vi "Untitled 1.vi"() -> ()   [LabVIEW 2021, in "FFT.lvlib"]
uses:
  FFT.lvlib
  <vilib>/Analysis/4window.llb/Hanning Window (DBL).vi
  <vilib>/Analysis/5stat.llb/RMS (DBL).vi
  <vilib>/Analysis/2dsp.llb/Real FFT.vi
  <vilib>/Analysis/4window.llb/AllCosWindow (DBL).vi
  <vilib>/Analysis/NI_AALPro.lvlib
panel:
  out "ACC Data":dbl[](array[numeric])
  out "Frequency measured":dbl
  out "FFT":dbl[](array[numeric])
  out "Low-Energy Warning":bool
  in  "Bound to 1st Frequency":bool=TRUE
  in  "Experiment":T1
  in  "Accelerometer sample":dbl[](array[numeric])
  in  "Frequency Method":T2(ring)
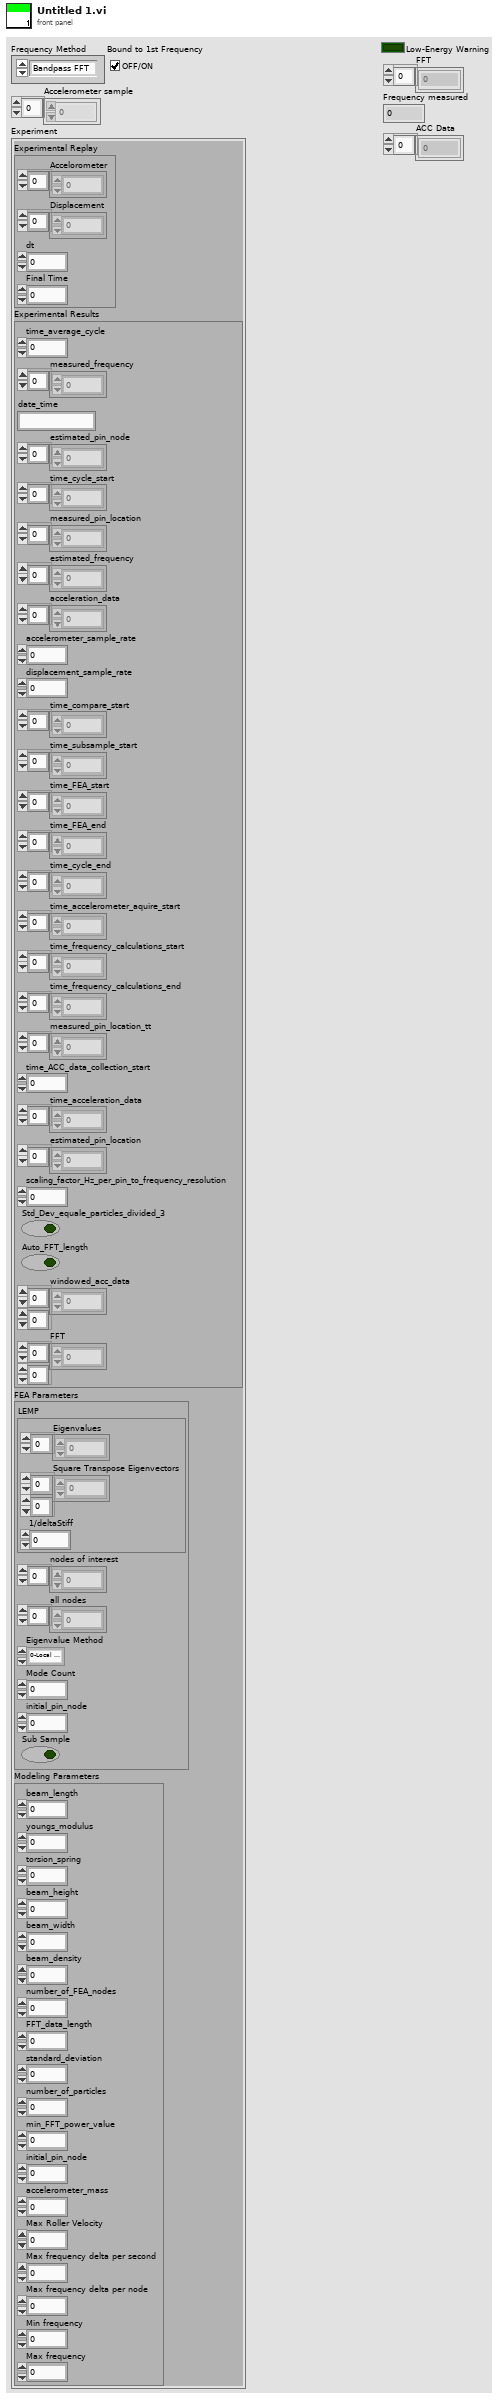
[diagram p1: front panel]
types:
  T1 = cluster{"Experimental Replay":cluster{"Accelorometer":dbl[], "Displacement":dbl[], "dt":dbl, "Final Time":dbl}, "Experimental Results":cluster{"time_average_cycle":dbl, "measured_frequency":dbl[], "date_time":string, "estimated_pin_node":i32[], "time_cycle_start":dbl[], "measured_pin_location":dbl[], "estimated_frequency":dbl[], "acceleration_data":dbl[], "accelerometer_sample_rate":dbl, "displacement_sample_rate":dbl, "time_compare_start":dbl[], "time_subsample_start":dbl[], "time_FEA_start":dbl[], "time_FEA_end":dbl[], "time_cycle_end":dbl[], "time_accelerometer_aquire_start":dbl[], "time_frequency_calculations_start":dbl[], "time_frequency_calculations_end":dbl[], "measured_pin_location_tt":dbl[], "time_ACC_data_collection_start":dbl, "time_acceleration_data":dbl[], "estimated_pin_location":dbl[], "scaling_factor_Hz_per_pin_to_frequency_resolution":dbl, "Std_Dev_equale_particles_divided_3":bool, "Auto_FFT_length":bool, "windowed_acc_data":dbl[][], "FFT":dbl[][]}, "FEA Parameters":cluster{"LEMP":cluster{"Eigenvalues":dbl[], "Square Transpose Eigenvectors":dbl[][], "1/deltaStiff":dbl}, "nodes of interest":i32[], "all nodes":i32[], "Eigenvalue Method":enum16{"0-Local Eigen Modification Procedure", "1-LabVIEW generalized eigenvalues", "2-LabVIEW M^-1K eigenvalues", "3-LabVIEW Cholesky Factorization", "4-Cholesky Factorization CPU SGL", "5-Cholesky Factorization CPU FXP", "6-Cholesky Factorization FPGA SGL", "7-Cholesky Factorization FPGA SGL SCL"}, "Mode Count":i32, "initial_pin_node":i32, "Sub Sample":bool}, "Modeling Parameters":cluster{"beam_length":dbl, "youngs_modulus":dbl, "torsion_spring":dbl, "beam_height":dbl, "beam_width":dbl, "beam_density":dbl, "number_of_FEA_nodes":i32, "FFT_data_length":i32, "standard_deviation":dbl, "number_of_particles":i32, "min_FFT_power_value":dbl, "initial_pin_node":i32, "accelerometer_mass":dbl, "Max Roller Velocity":dbl, "Max frequency delta per second":dbl, "Max frequency delta per node":dbl, "Min frequency":dbl, "Max frequency":dbl}}
  T2 = enum16{"Bandpass FFT", "Tone", "FFT", "Custom Filter"}
  T3 = cluster{"Frequency Method":enum16{"Bandpass FFT", "Tone", "FFT", "Custom Filter"}, "Sample Rate":dbl, "FFT Power Threshold":dbl, "Window":i32, "Max frequency delta per second":dbl}
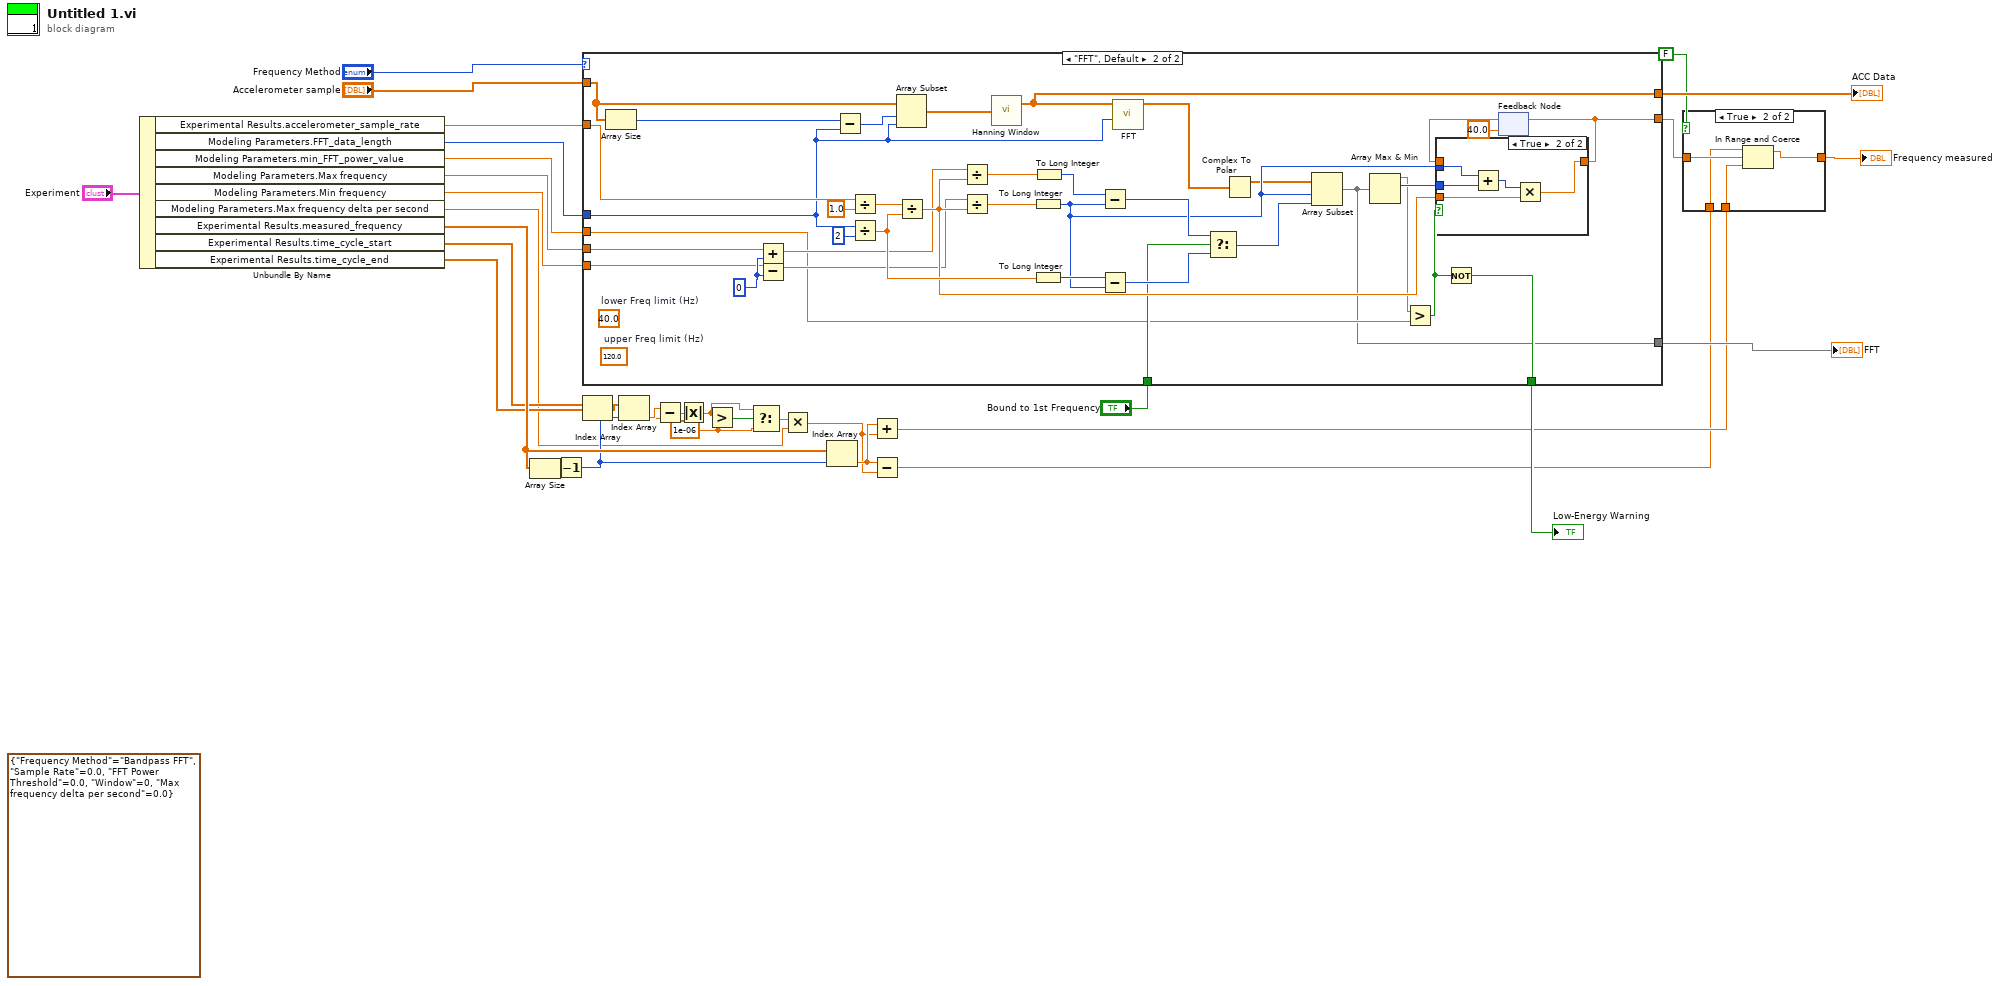
[diagram p0: block diagram]
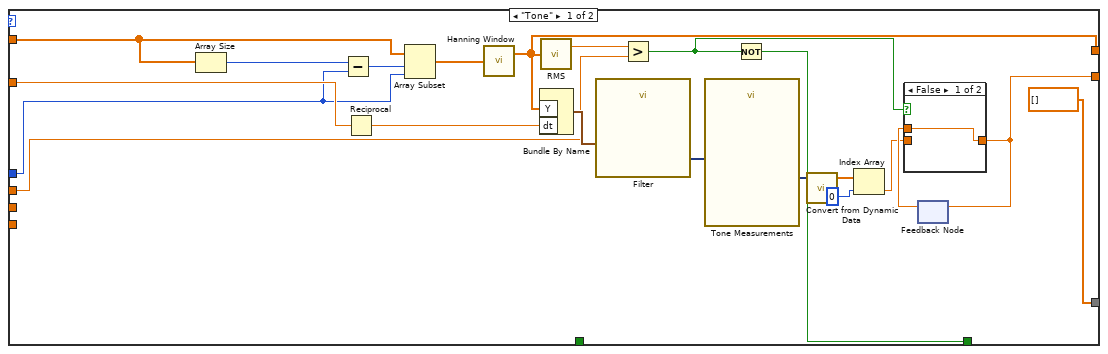
[diagram p3: hidden frame]
diagram:
  (unwired) T3 {"Frequency Method"=enum."Bandpass FFT", "Sample Rate"=0.0, "FFT Power Threshold"=0.0, "Window"=0, "Max frequency delta per second"=0.0}
  w4 = 1e-06 ("y")
  n1 = Unbundle By Name("Experiment") -> ("Experimental Results.accelerometer_sample_rate"=w29:dbl, "Modeling Parameters.FFT_data_length"=w25:i32, "Modeling Parameters.min_FFT_power_value"=w26:dbl, "Modeling Parameters.Max frequency"=w28:dbl, "Modeling Parameters.Min frequency"=w27:dbl, "Modeling Parameters.Max frequency delta per second"=w1:dbl, "Experimental Results.measured_frequency"=w18:dbl[], "Experimental Results.time_cycle_start"=w11:dbl[], "Experimental Results.time_cycle_end"=w10:dbl[])
  n2 = Array Size(array=w18) -> (size(s)=w17:i32)
  n3 = Decrement(x=w17) -> (x-1=w12:i32)
  n4 = case shown="\"FFT\", Default" "Frequency Method" {
    tunnel: [w41 w60] -> w20
    tunnel: [w43 w73] -> w21
    tunnel: "Accelerometer sample" -> [w45 w75]
    tunnel: [w38 w72] -> w23
    tunnel: "Bound to 1st Frequency" -> [_ w74]
    tunnel: [dbl[] [] ("Real freq comp (out)") w58] -> w22
    tunnel: w29 -> [w35 w64]
    tunnel: w28 -> [_ w61]
    tunnel: w27 -> [_ w56]
    tunnel: w26 -> [w33 w62]
    tunnel: w25 -> [w34 w63]
    frame "Tone" {
      n5 = Array Size(array=w45) -> (size(s)=w53:i32)
      n6 = Subtract(x=w53, y=w34) -> (x-y=w52:i32)
      n7 = Reciprocal(x=w35) -> (1/x=w37:dbl)
      n8 = Array Subset(array=w45, index=w52, length=w34) -> (w46:dbl[])
      n9 = call-poly <vilib>:"Hanning Window.vi"("X"=w46) -> ("Windowed X"=w43:dbl[])  [unwired: 1 out]
      n10 = Bundle By Name("Y"=w43, "dt"=w37) -> (w47:waveform(dbl))  [unwired: 1 in]
      n11 = call-poly <vilib>:"RMS.vi"("X"=w43) -> ("rms value"=w39:dbl)  [unwired: 1 out]
      n12 = call "Filter"("Signal"=w47) -> ("Filtered Signal"=w48:dynamicdata)  [unwired: 9 in, 1 out]
      n13 = Greater?(x=w39, y=w33) -> (0:w40:bool)
      n14 = call "Tone Measurements"("Signals"=w48) -> ("Frequency"=w49:dynamicdata)  [unwired: 9 in, 1 out]
      n15 = Not(x=w40) -> (.not. x?=w38:bool)
      n16 = call "Convert from Dynamic Data"("Dynamic Data Type"=w49) -> ("Array"=w50:dbl[])  [unwired: 3 in]
      n17 = Index Array(array=w50, index=0) -> (element=w42:dbl)
      n18 = feedback #1() -> (w44:dbl)  [unwired: 1 in]
      n19 = case shown="False" w40 {
        tunnel: [w54 w55] -> w41
        tunnel: w44 -> [w54 _]
        tunnel: w42 -> [_ w55]
        frame False {
        }
        frame True {
        }
      }
      n20 = feedback-in #1(w41) -> ()
    }
    frame "FFT", Default {
      w57 = 0
      (unwired) 120.0  # upper Freq limit (Hz)
      (unwired) 40.0  # lower Freq limit (Hz)
      n21 = Array Size(array=w75) -> (size(s)=w85:i32)
      n22 = Add(x=w61, y=w57) -> (x+y=w66:dbl)
      n23 = Subtract(x=w56, y=w57) -> (x-y=w67:dbl)
      n24 = Subtract(x=w85, y=w63) -> (x-y=w84:i32)
      n25 = Divide(x=w64, y=1.0) -> (x/y=w87:dbl)
      n26 = Divide(x=w63, y=2) -> (x/y=w86:dbl)
      n27 = Array Subset(array=w75, index=w84, length=w63) -> (w83:dbl[])
      n28 = Divide(x=w87, y=w86) -> (x/y=w81:dbl)
      n29 = Divide(x=w66, y=w81) -> (x/y=w80:dbl)
      n30 = Divide(x=w67, y=w81) -> (x/y=w91:dbl)
      n31 = call-poly <vilib>:"Hanning Window.vi"("X"=w83) -> ("Windowed X"=w73:dbl[])  [unwired: 1 out]
      n32 = To Long Integer(number=w91) -> (32bit integer=w68:i32)
      n33 = To Long Integer(number=w86) -> (32bit integer=w89:i32)
      n34 = To Long Integer(number=w80) -> (32bit integer=w79:i32)
      n35 = Subtract(x=w79, y=w68) -> (x-y=w77:i32)
      n36 = Subtract(x=w89, y=w68) -> (x-y=w76:i32)
      n37 = call-poly <vilib>:"FFT.vi"("FFT size"=w63, "X"=w73) -> ("FFT {X}"=w71:cdb[])  [unwired: 8 in, 1 out]
      n38 = Select(t=w77, s=w74, f=w76) -> (s? t:f=w78:i32)
      n39 = Complex To Polar(r * e^(i*theta)=w71) -> (r=w59:dbl[])  [unwired: 1 out]
      n40 = Array Subset(array=w59, index=w68, length=w78) -> (w58:dbl[])
      n41 = Array Max & Min(array=w58) -> (max value=w65:dbl, max index (indices)=w90:i32)  [unwired: 2 out]
      n42 = Greater?(x=w65, y=w62) -> (0:w82:bool)
      n43 = Not(x=w82) -> (.not. x?=w72:bool)
      n44 = feedback #2(40.0) -> (w70:dbl)
      n45 = case shown="True" w82 {
        tunnel: w90 -> [_ w95]
        tunnel: w68 -> [_ w96]
        tunnel: w81 -> [_ w97]
        tunnel: [w93 w94] -> w60
        tunnel: w70 -> [w93 _]
        frame False {
        }
        frame True {
          n46 = Add(x=w96, y=w95) -> (x+y=w98:i32)
          n47 = Multiply(x=w98, y=w97) -> (x*y=w94:dbl)
        }
      }
      n48 = feedback-in #2(w60) -> ()
    }
  }
  "Low-Energy Warning" <- w23
  "FFT" <- w22
  "ACC Data" <- w21
  n49 = Index Array(array=w11, index=w12) -> (element=w9:dbl)
  n50 = Index Array(array=w10, index=w12) -> (element=w8:dbl)
  n51 = Subtract(x=w9, y=w8) -> (x-y=w7:dbl)
  n52 = Absolute Value(x=w7) -> (abs(x)=w5:dbl)
  n53 = Greater?(x=w5, y=w4) -> (0:w6:bool)
  n54 = Select(t=w5, s=w6, f=w4) -> (s? t:f=w3:dbl)
  n55 = Multiply(x=w3, y=w1) -> (x*y=w2:dbl)
  n56 = Index Array(array=w18, index=w12) -> (element=w16:dbl)
  n57 = Add(x=w16, y=w2) -> (x+y=w15:dbl)
  n58 = Subtract(x=w16, y=w2) -> (x-y=w14:dbl)
  n59 = case shown="True" FALSE {
    tunnel: w20 -> [w99 w103]
    tunnel: [w99 w102] -> w19
    tunnel: w15 -> [_ w100]
    tunnel: w14 -> [_ w101]
    frame False {
    }
    frame True {
      n60 = In Range and Coerce(upper limit=w101, x=w103, lower limit=w100) -> (coerced(x)=w102:dbl)  [unwired: 1 out]
    }
  }
  "Frequency measured" <- w19
